vi "pp3_DAQ_AudioLoadImpl.vi"(5 "Daq config In":T1={"Sound AO"="Dev6/ao0", "Shock intesity AO"="Dev6/ao1", "Code_LED DO"="Dev6/port1:2", "Switch DI"="Dev6/port1/line0", "Webcam"="cam9", "Sound AO task"="", "Sound card task"=0, "Shock intensity AO task"="", "Code_LED DO task"="", "Switch DI task"="", "AO <=> Sound card"=FALSE, "Sound card"=0, "sample rate"=100000.0, "Variable shock"=TRUE, "Webcam on"=FALSE, "Waveform memo"={"t0"=timestamp(0 s since 1904-01-01), "dt"=1.0, "Y"=[]}, "First time"=FALSE, "Tone trigger"="", "Master-9 DO"="Dev6/port0/line5:7"} {"sample rate" min=8000.0; "Sound card task" format="%.0x"}, 7 "Waveform":waveform(dbl), 11 "error in (no error)":errorcluster) -> (6 "Daq config Out":T1={"Sound AO"="Dev6/ao0", "Shock intesity AO"="Dev6/ao1", "Code_LED DO"="Dev6/port1:2", "Switch DI"="Dev6/port1/line0", "Webcam"="cam9", "Sound AO task"="", "Sound card task"=0, "Shock intensity AO task"="", "Code_LED DO task"="", "Switch DI task"="", "AO <=> Sound card"=FALSE, "Sound card"=0, "sample rate"=100000.0, "Variable shock"=TRUE, "Webcam on"=FALSE, "Waveform memo"={"t0"=timestamp(0 s since 1904-01-01), "dt"=1.0, "Y"=[]}, "First time"=FALSE, "Tone trigger"="", "Master-9 DO"="Dev6/port0/line5:7"} {"sample rate" min=8000.0; "Sound card task" format="%.0x"}, 15 "error out":errorcluster)   [LabVIEW 2013]
uses:
  pp3_CTL_DaqConfig.ctl
  <vilib>/userdefined/High Color/IMAQdx.ctl
  <vilib>/sound2/lvsound2.llb/Sound Output Task ID.ctl
  <vilib>/DAQmx/write.llb/DAQmx Write (Analog Wfm 1Chan NSamp).vi
  <vilib>/DAQmx/create/channels.llb/DAQmx Create Channel (AO-Voltage-Basic).vi
  <vilib>/DAQmx/configure/timing.llb/DAQmx Timing (Use Waveform).vi
  <vilib>/DAQmx/miscellaneous.llb/DAQmx Fill In Error Info.vi
  <resource>/objmgr/daqmx.rc
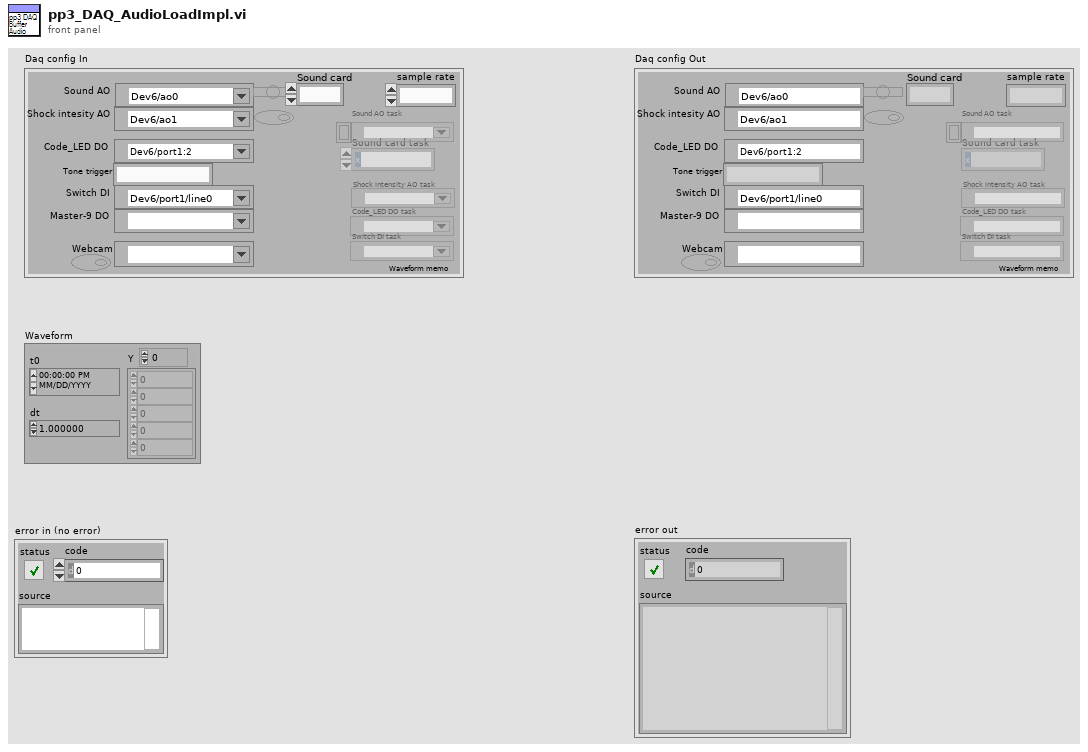
[diagram p1: front panel]
types:
  T1 = typedef "pp3_CTL_DaqConfig.ctl" = cluster{"Sound AO":tag, "Shock intesity AO":tag, "Code_LED DO":tag, "Switch DI":tag, "Webcam":T2, "Sound AO task":refnum<k21>, "Sound card task":T3, "Shock intensity AO task":refnum<k21>, "Code_LED DO task":refnum<k21>, "Switch DI task":refnum<k21>, "AO <=> Sound card":bool, "Sound card":u32, "sample rate":dbl, "Variable shock":bool, "Webcam on":bool, "Waveform memo":waveform(dbl), "First time":bool, "Tone trigger":string, "Master-9 DO":tag}
  T2 = typedef "IMAQdx.ctl" = refnum<k21>
  T3 = typedef "Sound Output Task ID.ctl" = u32
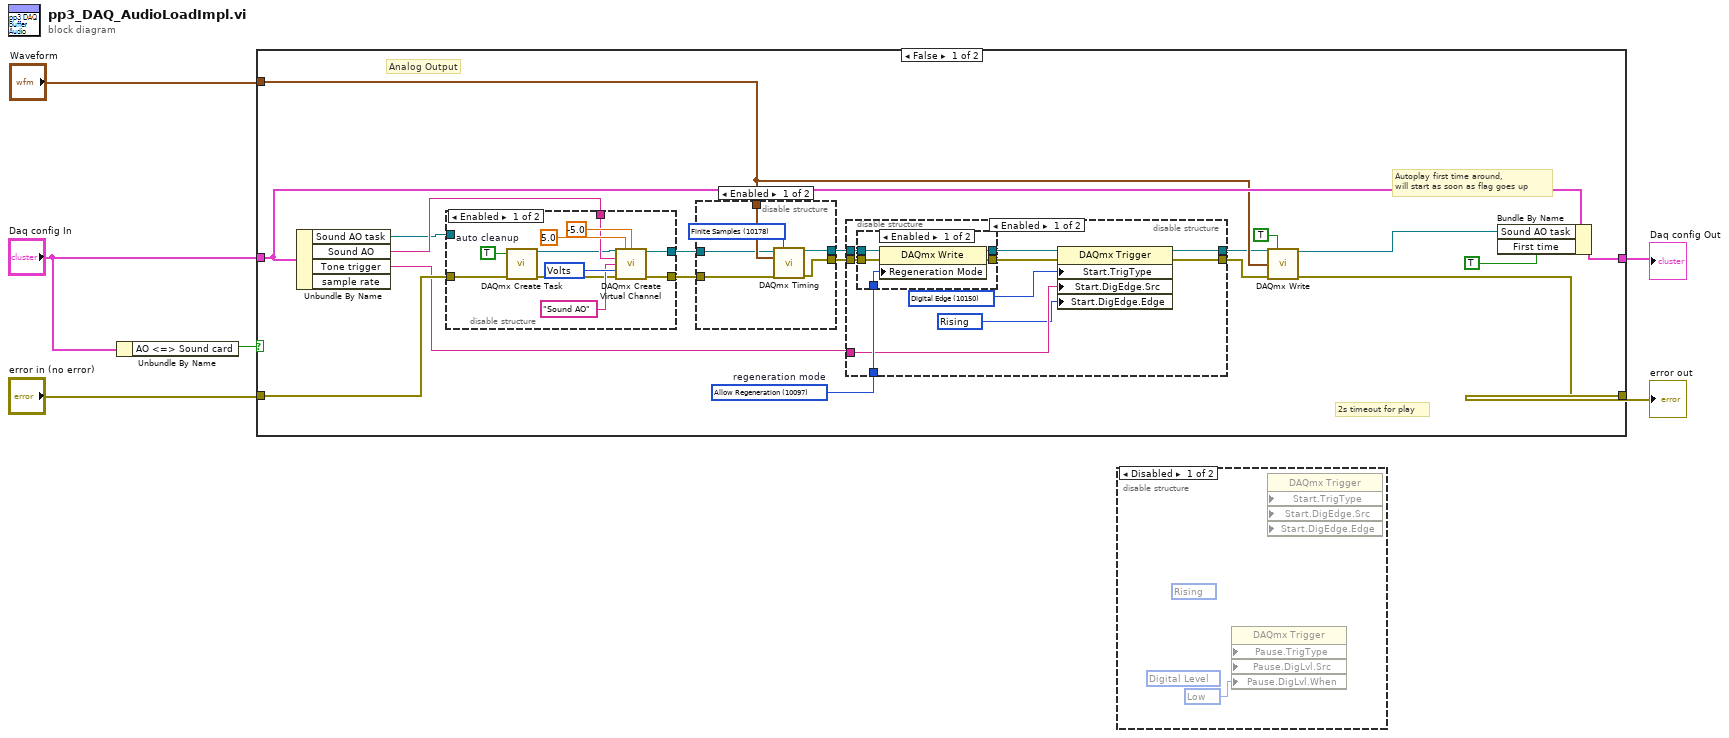
[diagram p0: block diagram]
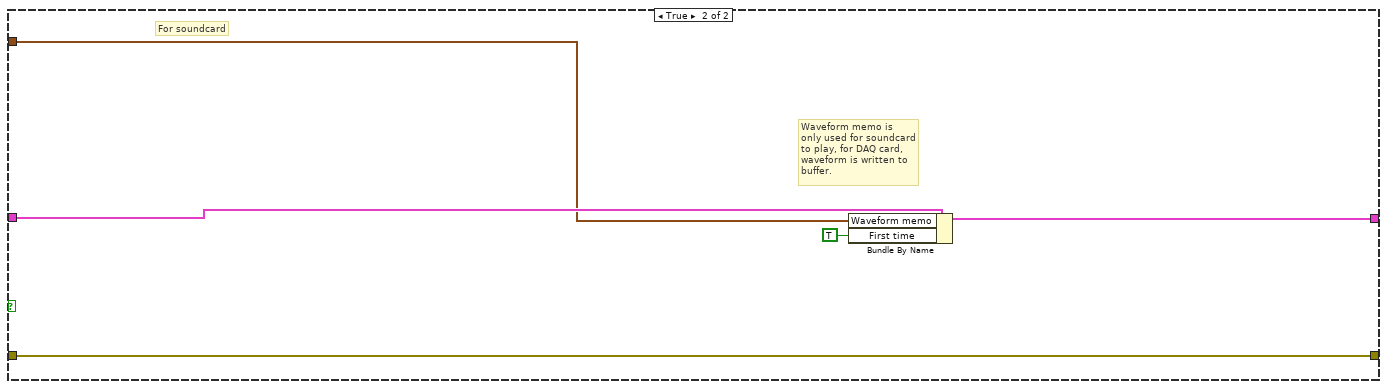
[diagram p7: hidden frame]
diagram:
  n1 = Unbundle By Name("Daq config In") -> ("AO <=> Sound card"=w6:bool)
  n2 = case shown="False" w6 {
    tunnel: "Daq config In" -> [w23 w68]
    tunnel: [w22 w69] -> w3
    tunnel: "error in (no error)" -> [w15 w66]
    tunnel: [w7 w66] -> w2
    tunnel: "Waveform" -> [w21 w67]
    frame False {
      w16 = 10097 items=["Allow Regeneration"=10097, "Do Not Allow Regeneration"=10158]  # regeneration mode
      # "2s timeout for play"
      # "Autoplay first time around,\nwill start as soon as flag goes up"
      # "Analog Output"
      n3 = Unbundle By Name(w23) -> ("Sound AO task"=w10:refnum<k21>, "Sound AO"=w18:tag, "Tone trigger"=w12:string)  [unwired: 1 out]
      n4 = disable-structure shown="Enabled" {
        disable-tunnel: [w39 w45] -> w20
        disable-tunnel: [w38 w44] -> w19
        disable-tunnel: w18 -> [w37 _]
        disable-tunnel: w15 -> [w34 w44]
        disable-tunnel: w10 -> [_ w45]
        frame Enabled {
          w36 = TRUE  # auto cleanup
          w43 = 10348 items=["Volts"=10348, "From Custom Scale"=10065] ("units")
          n5 = call <vilib>:"DAQmx Create Task.vi"("auto cleanup"=w36, "error in"=w34) -> ("task out"=w35:refnum<k21>, "error out"=w33:errorcluster)  [unwired: 12 in]
          n6 = call-poly <vilib>:"DAQmx Create Virtual Channel.vi"("task in"=w35, "maximum value"=5.0, "minimum value"=-5.0, "physical channels"=w37, "name to assign"="Sound AO", "units"=w43, "error in"=w33) -> ("task out"=w39:refnum<k21>, "error out"=w38:errorcluster)  [unwired: 7 in]
        }
        frame Disabled {
        }
      }
      n7 = disable-structure shown="Enabled" {
        disable-tunnel: w21 -> [w29 _]
        disable-tunnel: w20 -> [w28 w32]
        disable-tunnel: w19 -> [w27 w31]
        disable-tunnel: [w26 w31] -> w17
        disable-tunnel: [w25 w32] -> w9
        frame Enabled {
          w30 = 10178 items=["Finite Samples"=10178, "Continuous Samples"=10123, "Hardware Timed Single Point"=12522] ("sample mode")
          n8 = call-poly <vilib>:"DAQmx Timing.vi"("task/channels in"=w28, "sample mode"=w30, "waveform"=w29, "error in"=w27) -> ("task out"=w25:refnum<k21>, "error out"=w26:errorcluster)  [unwired: 10 in]
        }
        frame Disabled {
        }
      }
      n9 = disable-structure shown="Enabled" {
        disable-tunnel: w9 -> [w55 w64]
        disable-tunnel: w17 -> [w54 w63]
        disable-tunnel: w16 -> [w53 _]
        disable-tunnel: [w49 w64] -> w14
        disable-tunnel: [w48 w63] -> w13
        disable-tunnel: w12 -> [w50 _]
        frame Enabled {
          w47 = 10150 items=["Analog Edge"=10099, "Digital Edge"=10150, "Digital Pattern"=10398, "Analog Window"=10103, "None"=10230] ("Start.TrigType")
          w46 = 10280 items=["Rising"=10280, "Falling"=10171] ("Start.DigEdge.Edge")
          n10 = disable-structure shown="Enabled" {
            disable-tunnel: w55 -> [w60 w62]
            disable-tunnel: w54 -> [w59 w61]
            disable-tunnel: w53 -> [w58 _]
            disable-tunnel: [w57 w62] -> w52
            disable-tunnel: [w56 w61] -> w51
            frame Enabled {
              n11 = property class="DAQmx Write"(reference=w60, error in=w59, "Regeneration Mode"=w58) -> (reference out=w57:refnum<k21>, error out=w56:errorcluster)
            }
            frame Disabled {
            }
          }
          n12 = property class="DAQmx Trigger"(reference=w52, error in=w51, "Start.TrigType"=w47, "Start.DigEdge.Src"=w50, "Start.DigEdge.Edge"=w46) -> (reference out=w49:refnum<k21>, error out=w48:errorcluster)
        }
        frame Disabled {
        }
      }
      n13 = call-poly <vilib>:"DAQmx Write.vi"("task/channels in"=w14, "auto start"=TRUE, "data"=w21, "error in"=w13) -> ("task out"=w8:refnum<k21>, "error out"=w7:errorcluster)  [unwired: 9 in, 1 out]
      n14 = Bundle By Name(cluster=w23, "Sound AO task"=w8, "First time"=TRUE) -> (w22:T1)
    }
    frame True {
      # "For soundcard"
      # "Waveform memo is\nonly used for soundcard\nto play, for DAQ card,\nwaveform is written to\nbuffer."
      n15 = Bundle By Name(cluster=w68, "Waveform memo"=w67, "First time"=TRUE) -> (w69:T1)
    }
  }
  "Daq config Out" <- w3
  "error out" <- w2
  n16 = disable-structure shown="Disabled" {
    frame Disabled {
      w70 = 10214 items=["High"=10192, "Low"=10214] ("Pause.DigLvl.When")
      (unwired) 10152 items=["Analog Level"=10101, "Analog Window"=10103, "Digital Level"=10152, "Digital Pattern"=10398, "None"=10230] ("Pause.TrigType")
      (unwired) 10280 items=["Rising"=10280, "Falling"=10171] ("Start.DigEdge.Edge")
      n17 = property class="DAQmx Trigger" props=["Pause.TrigType", "Pause.DigLvl.Src", "Pause.DigLvl.When"]("Pause.DigLvl.When"=w70) -> ()  [unwired: 4 in, 2 out]
      n18 = property class="DAQmx Trigger" props=["Start.TrigType", "Start.DigEdge.Src", "Start.DigEdge.Edge"]() -> ()  [unwired: 5 in, 2 out]
    }
    frame Enabled {
    }
  }
